vi "Open Generic Property.vi"(0 "SLSC Remote in":refnum<class "SLSC Remote.lvclass">, 5 "resource":string, 7 "property in":refnum<k21>, 11 "error in (no error)":errorcluster) -> (4 "SLSC Remote out":refnum<class "SLSC Remote.lvclass">, 8 "property out":refnum<k21>, 15 "error out":errorcluster)   [LabVIEW 2016, in "SLSC Interfaces.lvlib" / "SLSC Remote.lvclass"]
uses:
  SLSC Remote.lvclass
  C:/Users/tblair/Documents/SLSC-Interface/Source/SLSC Interface Class/SLSC Interface.lvclass
  <vilib>/rajsite/i3-json/JSON Generation/Create Value Files/Create Value - Object.vi
  <vilib>/rajsite/i3-json/JSON Generation/Add Object Parameter Files/Add Object Parameter - String.vi
  <vilib>/NI/NI JSONRPC Server Framework/Classes/Server/Format Client Request (Auto-Increment).vi
  <vilib>/httpClient/POSTBuffer.vi
  <vilib>/NI/NI JSONRPC Server Framework/Classes/Server/JSONRPC Server.lvclass
  <vilib>/rajsite/i3-json/i3-json.lvlib
  <vilib>/httpClient/LabVIEWHTTPClient.lvlib
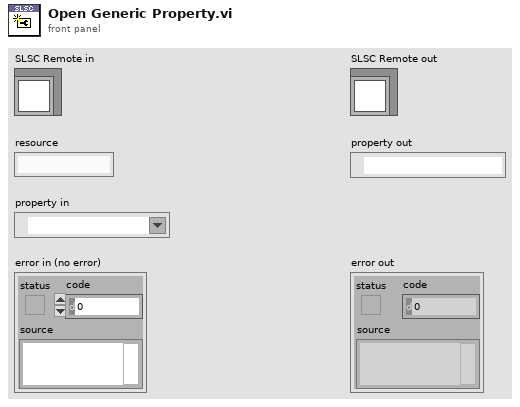
[diagram p1: front panel]
types:
  T1 = typedef "LabVIEWHTTPClient.lvlib/ClientHandle.ctl" = refnum<k1>
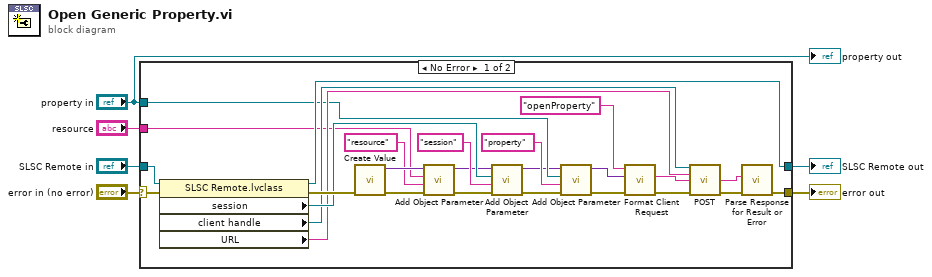
[diagram p0: block diagram]
diagram:
  n1 = case shown="No Error" "error in (no error)" {
    selector: "error in (no error)" -> [w30 w33]
    tunnel: "property in" -> [w18 _]
    tunnel: "SLSC Remote in" -> [w32 w34]
    tunnel: [w31 w34] -> w5
    tunnel: [w20 w33] -> w3
    tunnel: "resource" -> [w7 _]
    frame No Error {
      n2 = property class="SLSC Remote.lvclass"(reference=w32, error in=w30) -> (reference out=w31:refnum<class "SLSC Remote.lvclass">, error out=w29:errorcluster, "session"=w27:refnum<k21>, "client handle"=w25:T1, "URL"=w24:string)
      n3 = call-poly <vilib>:"Create Value.vi"("error in (no error)"=w29) -> ("error out"=w11:errorcluster, "JSON Tree"=w12:variant)  [unwired: 9 in]
      n4 = call-poly <vilib>:"Add Object Parameter.vi"("error in (no error)"=w11, "Name"="resource", "String"=w7, "JSON Tree in (JSON Object)"=w12) -> ("error out"=w9:errorcluster, "JSON Tree out (JSON Object)"=w10:variant)  [unwired: 6 in]
      n5 = call-poly <vilib>:"Add Object Parameter.vi"("error in (no error)"=w9, "Name"="session", "String"=w27, "JSON Tree in (JSON Object)"=w10) -> ("error out"=w16:errorcluster, "JSON Tree out (JSON Object)"=w17:variant)  [unwired: 6 in]
      n6 = call-poly <vilib>:"Add Object Parameter.vi"("error in (no error)"=w16, "Name"="property", "String"=w18, "JSON Tree in (JSON Object)"=w17) -> ("error out"=w14:errorcluster, "JSON Tree out (JSON Object)"=w15:variant)  [unwired: 6 in]
      n7 = call-poly <vilib>:"Format Client Request.vi"("error in (no error)"=w14, "params"=w15, "method"="openProperty") -> ("error out"=w23:errorcluster, "Request String"=w28:string)  [unwired: 7 in]
      n8 = call-poly <vilib>:"POST.vi"("client handle"=w25, "url"=w24, "buffer"=w28, "error in (no error)"=w23) -> ("body"=w22:string, "error out"=w21:errorcluster)  [unwired: 8 in, 2 out]
      n9 = call <vilib>:"Parse Response for Result or Error.vi"("error in"=w21, "Response String In"=w22) -> ("error out"=w20:errorcluster)  [unwired: 7 in, 2 out]
    }
    frame Error {
    }
  }
  "error out" <- w3
  "SLSC Remote out" <- w5
  "property out" <- "property in"
